vi "gameplay scene.vi"(8 "hold note key":T1, 9 "gameplay info":T2, 10 "chart info":T3, 11 "new picture in":picture) -> (3 "new picture":picture)   [LabVIEW 2023]
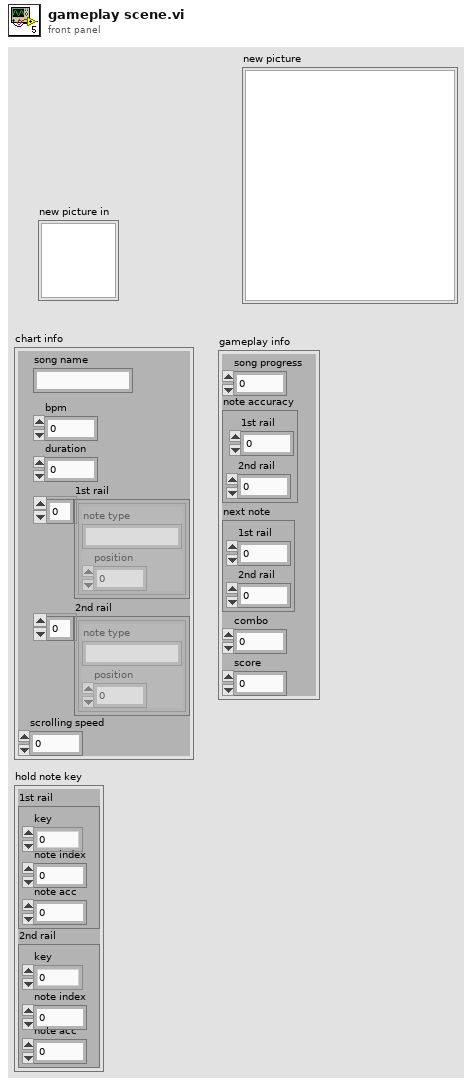
[diagram p1: front panel]
types:
  T1 = cluster{"1st rail":cluster{"key":enum16{"0", "1", "2", "3", "4", "5", "6", "7", "8", "9", "A", "B", "C", "D", "E", "F", "G", "H", "I", "J", "K", "L", "M", "N", "O", "P", "Q", "R", "S", "T", "U", "V", "W", "X", "Y", "Z", "F1", "F2", "F3", "F4", "F5", "F6", "F7", "F8", "F9", "F10", "F11", "F12", "F13", "F14", "F15", "ADD", "BACK", "BACKSLASH", "CAPITAL", "COMMA", "DECIMAL", "DELETE", "DIVIDE", "DOWN", "END", "EQUALS", "ESCAPE", "GRAVE (`)", "HOME", "INSERT", "LBRACKET", "LCONTROL", "LEFT", "L ALT", "LSHIFT", "LWIN", "MINUS", "MULTIPLY", "NEXT", "NUMLOCK", "NUMPAD_0", "NUMPAD_1", "NUMPAD_2", "NUMPAD_3", "NUMPAD_4", "NUMPAD_5", "NUMPAD_6", "NUMPAD_7", "NUMPAD_8", "NUMPAD_9", "PAUSE", "PERIOD", "PRIOR (PG UP)", "RBRACKET", "RCONTROL", "RETURN", "RIGHT", "R ALT", "RSHIFT", "RWIN", "SCROLL", "SEMICOLON", "SLASH", "SPACE", "SUBTRACT", "TAB", "UP", "ENTER (num pad)", "' (quote)"}, "note index":i32, "note acc":i32}, "2nd rail":cluster{"key":enum16{"0", "1", "2", "3", "4", "5", "6", "7", "8", "9", "A", "B", "C", "D", "E", "F", "G", "H", "I", "J", "K", "L", "M", "N", "O", "P", "Q", "R", "S", "T", "U", "V", "W", "X", "Y", "Z", "F1", "F2", "F3", "F4", "F5", "F6", "F7", "F8", "F9", "F10", "F11", "F12", "F13", "F14", "F15", "ADD", "BACK", "BACKSLASH", "CAPITAL", "COMMA", "DECIMAL", "DELETE", "DIVIDE", "DOWN", "END", "EQUALS", "ESCAPE", "GRAVE (`)", "HOME", "INSERT", "LBRACKET", "LCONTROL", "LEFT", "L ALT", "LSHIFT", "LWIN", "MINUS", "MULTIPLY", "NEXT", "NUMLOCK", "NUMPAD_0", "NUMPAD_1", "NUMPAD_2", "NUMPAD_3", "NUMPAD_4", "NUMPAD_5", "NUMPAD_6", "NUMPAD_7", "NUMPAD_8", "NUMPAD_9", "PAUSE", "PERIOD", "PRIOR (PG UP)", "RBRACKET", "RCONTROL", "RETURN", "RIGHT", "R ALT", "RSHIFT", "RWIN", "SCROLL", "SEMICOLON", "SLASH", "SPACE", "SUBTRACT", "TAB", "UP", "ENTER (num pad)", "' (quote)"}, "note index":i32, "note acc":i32}}
  T2 = cluster{"song progress":dbl, "note accuracy":cluster{"1st rail":i32, "2nd rail":i32}, "next note":cluster{"1st rail":i32, "2nd rail":i32}, "combo":i32, "score":i32}
  T3 = cluster{"song name":string, "bpm":i32, "duration":i32, "1st rail":cluster{"note type":string, "position":dbl}[], "2nd rail":cluster{"note type":string, "position":dbl}[], "scrolling speed":dbl}
  T4 = cluster{"Font Name:":string, "Size":i16, "Strikeout?":bool, "Italic?":bool, "Underline?":bool, "Outline?":bool, "Shadow?":bool, "Bold?":bool}
  T5 = enum16{"User-specified Font", "Application Font", "System Font", "Dialog Font"}
  T6 = cluster{"horizontal":enum16{"left", "center", "right"}, "vertical":enum16{"top", "center", "bottom"}}
  T7 = enum16{"0", "1", "2", "3", "4", "5", "6", "7", "8", "9", "A", "B", "C", "D", "E", "F", "G", "H", "I", "J", "K", "L", "M", "N", "O", "P", "Q", "R", "S", "T", "U", "V", "W", "X", "Y", "Z", "F1", "F2", "F3", "F4", "F5", "F6", "F7", "F8", "F9", "F10", "F11", "F12", "F13", "F14", "F15", "ADD", "BACK", "BACKSLASH", "CAPITAL", "COMMA", "DECIMAL", "DELETE", "DIVIDE", "DOWN", "END", "EQUALS", "ESCAPE", "GRAVE (`)", "HOME", "INSERT", "LBRACKET", "LCONTROL", "LEFT", "L ALT", "LSHIFT", "LWIN", "MINUS", "MULTIPLY", "NEXT", "NUMLOCK", "NUMPAD_0", "NUMPAD_1", "NUMPAD_2", "NUMPAD_3", "NUMPAD_4", "NUMPAD_5", "NUMPAD_6", "NUMPAD_7", "NUMPAD_8", "NUMPAD_9", "PAUSE", "PERIOD", "PRIOR (PG UP)", "RBRACKET", "RCONTROL", "RETURN", "RIGHT", "R ALT", "RSHIFT", "RWIN", "SCROLL", "SEMICOLON", "SLASH", "SPACE", "SUBTRACT", "TAB", "UP", "ENTER (num pad)", "' (quote)"}
  T8 = cluster{"Width":u16, "Style":enum32{"Solid", "Dash", "Dot", "DashDot", "DashDotDot"}}
  T9 = cluster{"Width":i16, "Style":enum32{"Solid", "Dash", "Dot", "DashDot", "DashDotDot"}}
  T10 = enum16{"0", "1", "2", "3", "4", "5", "6", "7", "8", "9", "A", "B", "C", "D", "E", "F", "G", "H", "I", "J", "K", "L", "M", "N", "O", "P", "Q", "R", "S", "T", "U", "V", "W", "X", "Y", "Z", "F1", "F2", "F3", "F4", "F5", "F6", "F7", "F8", "F9", "F10", "F11", "F12", "F13", "F14", "F15", "ADD", "BACK", "BACKSLASH", "CAPITAL", "COMMA", "DECIMAL", "DELETE", "DIVIDE", "DOWN", "END", "EQUALS", "ESCAPE", "GRAVE (`)", "HOME", "INSERT", "LBRACKET", "LCONTROL", "LEFT", "L ALT", "LSHIFT", "LWIN", "MINUS", "MULTIPLY", "NEXT", "NUMLOCK", "NUMPAD_0", "NUMPAD_1", "NUMPAD_2", "NUMPAD_3", "NUMPAD_4", "NUMPAD_5", "NUMPAD_6", "NUMPAD_7", "NUMPAD_8", "NUMPAD_9", "PAUSE", "PERIOD", "PRIOR (PG UP)", "RBRACKET", "RCONTROL", "RETURN", "RIGHT", "R ALT", "RSHIFT", "RWIN", "SCROLL", "SEMICOLON", "SLASH", "SPACE", "SUBTRACT", "TAB", "UP", "ENTER (num pad)", "' (quote)"}[]
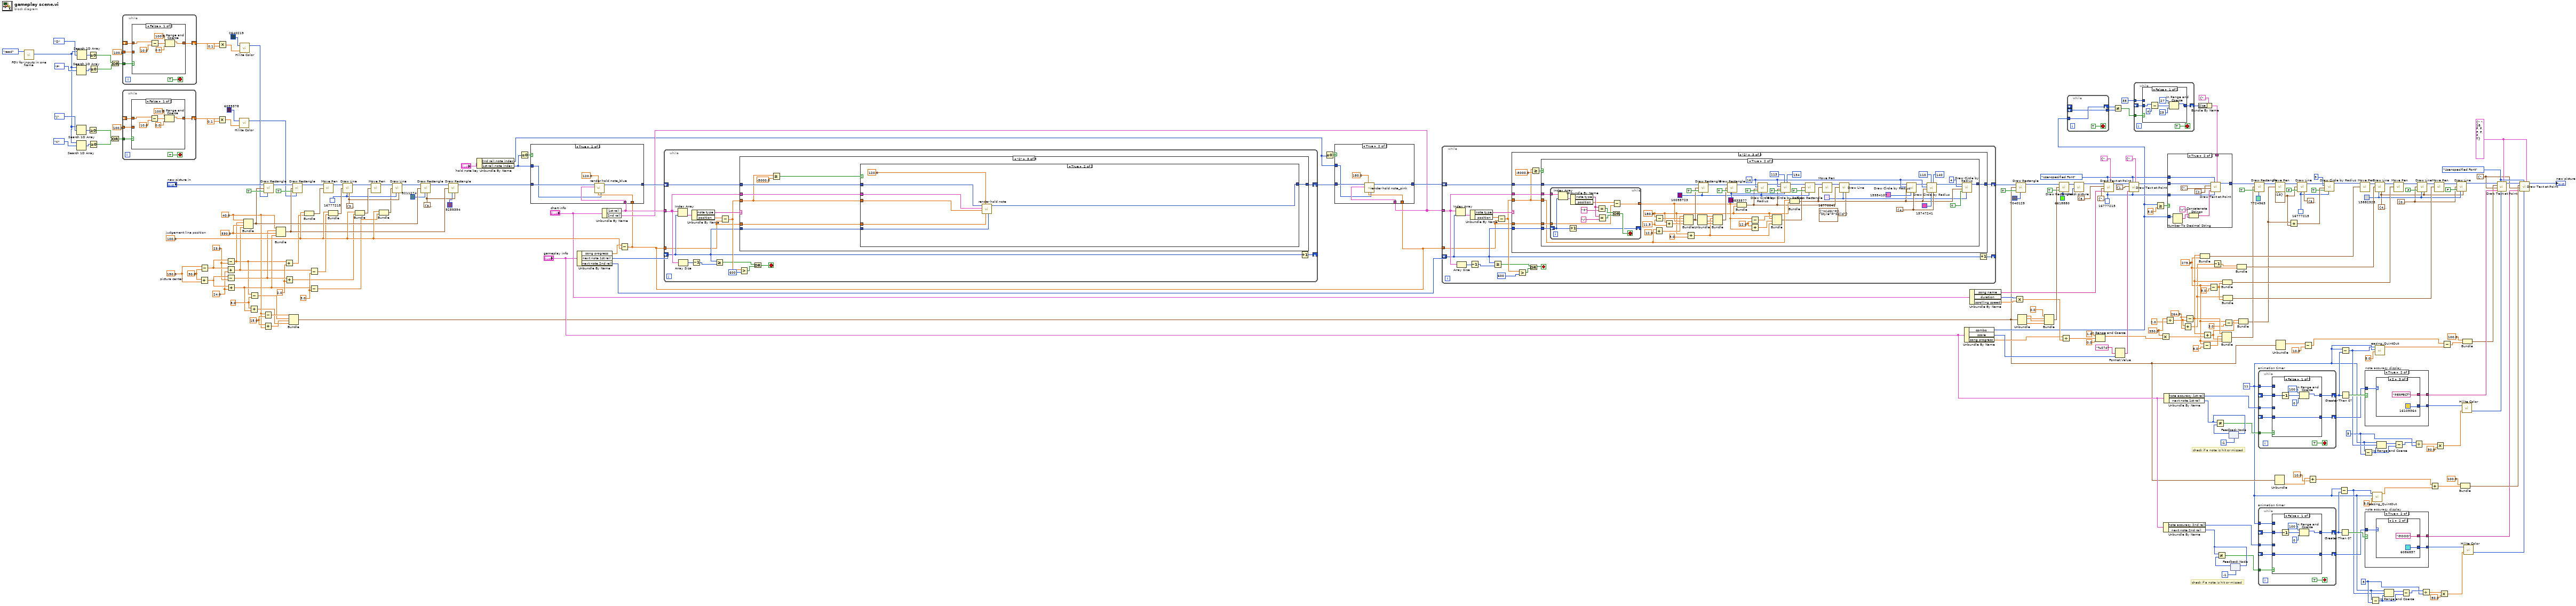
[diagram p0: block diagram]
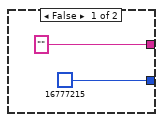
[diagram p2: hidden frame]
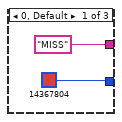
[diagram p3: hidden frame]
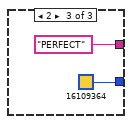
[diagram p4: hidden frame]
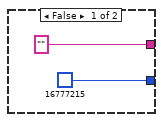
[diagram p6: hidden frame]
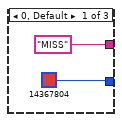
[diagram p7: hidden frame]
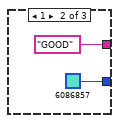
[diagram p8: hidden frame]
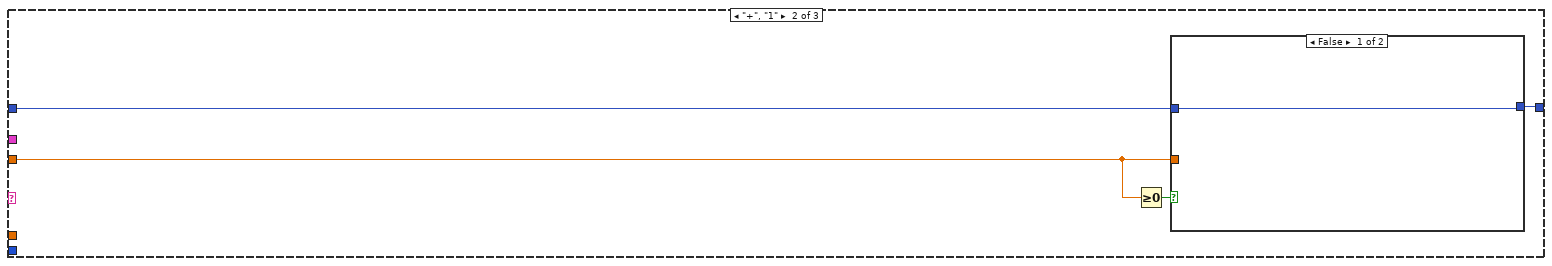
[diagram p17: hidden frame]
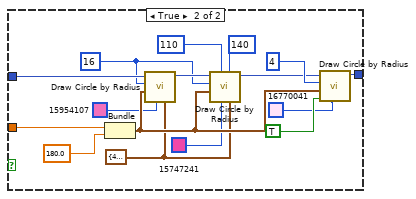
[diagram p18: hidden frame]
diagram:
  w12 = 5
  w39 = 5
  w9 = 11
  w19 = T4 {"Font Name:"=" ", "Size"=18, "Strikeout?"=FALSE, "Italic?"=FALSE, "Underline?"=FALSE, "Outline?"=FALSE, "Shadow?"=FALSE, "Bold?"=TRUE} ("[user-specified font]")
  w20 = T5."User-specified Font" ("desired font(Application)")
  w7 = T6 {"horizontal"=enum."center", "vertical"=enum."center"} ("alignment(left, top)")
  w115 = u32 16777215 ("color(black)")
  w119 = cluster{"x":i16, "y":i16} {"x"=0, "y"=-15} ("end point")
  w139 = cluster{"x":i16, "y":i16} {"x"=0, "y"=12} ("end point")
  w146 = u32 13882323 ("color(black)")
  w138 = T8 {"Width"=4, "Style"=enum."Solid"} ("pen")
  w129 = 275.0
  w160 = 264.0
  w162 = 350.0
  w167 = u32 16777215 ("text color(black)")
  w168 = T5."User-specified Font" ("desired font(Application)")
  w188 = u32 6618880 ("color(black)")
  w201 = 8.0
  w205 = 15.0
  w206 = 24.0
  w207 = 2.0
  w211 = 3.0
  w216 = T9 {"Width"=3, "Style"=enum."Solid"} ("pen")
  w222 = 530.0
  w214 = 23.0
  w228 = 30.0
  w227 = 150.0  # picture center
  w204 = 40.0
  w234 = T8 {"Width"=3, "Style"=enum."Solid"} ("pen")
  w233 = u32 16777215 ("color(black)")
  w231 = 100.0  # judgement line position
  # "check if a note is hit or missed"
  # "check if a note is hit or missed"
  n1 = call "FGV for inputs in one frame.vi"("mode"=enum16{"read", "write"}."read") -> ("read out key"=w74:T10)  [unwired: 10 in]
  n2 = Search 1D Array(1D array=w74, element=T7."K") -> (index of element=w76:i32)  [unwired: 1 in]
  n3 = Search 1D Array(1D array=w74, element=T7."F") -> (index of element=w99:i32)  [unwired: 1 in]
  n4 = Search 1D Array(1D array=w74, element=T7."J") -> (index of element=w75:i32)  [unwired: 1 in]
  n5 = Search 1D Array(1D array=w74, element=T7."D") -> (index of element=w100:i32)  [unwired: 1 in]
  n6 = Greater Or Equal To 0?(x=w75) -> (x >= 0?=w84:bool)
  n7 = Greater Or Equal To 0?(x=w100) -> (x >= 0?=w87:bool)
  n8 = Greater Or Equal To 0?(x=w76) -> (x >= 0?=w85:bool)
  n9 = Greater Or Equal To 0?(x=w99) -> (x >= 0?=w86:bool)
  n10 = Or(x=w84, y=w85) -> (x .or. y?=w83:bool)
  n11 = Or(x=w87, y=w86) -> (x .or. y?=w88:bool)
  n12 = while {
    tunnel: w83 -> [w247]
    tunnel: 100.0 -> [w246]
    shift-right: [w245] -> w78
    shift-left: _ -> [w244]
    stop <- TRUE stop-if-true
    n13 = case shown="False" w247 {
      tunnel: w246 -> [_ w255]
      tunnel: [w250 w255] -> w245
      tunnel: w244 -> [w254 _]
      frame False {
        n14 = Subtract(x=w254, y=10.0) -> (x-y=w252:dbl)
        n15 = In Range and Coerce(upper limit=100.0, x=w252, lower limit=0.0 ("upper limit")) -> (coerced(x)=w250:dbl)  [unwired: 1 out]
      }
      frame True {
      }
    }
  }
  n16 = while {
    tunnel: w88 -> [w259]
    tunnel: 100.0 -> [w258]
    shift-right: [w257] -> w97
    shift-left: _ -> [w256]
    stop <- TRUE stop-if-true
    n17 = case shown="False" w259 {
      tunnel: w258 -> [_ w267]
      tunnel: [w262 w267] -> w257
      tunnel: w256 -> [w266 _]
      frame False {
        n18 = Subtract(x=w266, y=10.0) -> (x-y=w264:dbl)
        n19 = In Range and Coerce(upper limit=100.0, x=w264, lower limit=0.0 ("upper limit")) -> (coerced(x)=w262:dbl)  [unwired: 1 out]
      }
      frame True {
      }
    }
  }
  n20 = Add(x=w228, y=w227) -> (x+y=w225:dbl)
  n21 = Subtract(x=w227, y=w228) -> (x-y=w226:dbl)
  n22 = Multiply(x=w78, y=0.1) -> (x*y=w80:dbl)
  n23 = Multiply(x=w97, y=0.1) -> (x*y=w95:dbl)
  n24 = Subtract(x=w226, y=w214) -> (x-y=w196:dbl)
  n25 = Add(x=w226, y=w206) -> (x+y=w200:dbl)
  n26 = Subtract(x=w225, y=w214) -> (x-y=w209:dbl)
  n27 = Add(x=w225, y=w206) -> (x+y=w199:dbl)
  n28 = call <vilib>:"Hilite Color.vi"("Percentage(30)"=w80, "Color In"=u32 6039378 ("color(black)")) -> ("Hilite"=w72:u32)  [unwired: 1 out]
  n29 = call <vilib>:"Hilite Color.vi"("Percentage(30)"=w95, "Color In"=u32 2640219 ("color(black)")) -> ("Hilite"=w92:u32)  [unwired: 1 out]
  n30 = Bundle(w204, w196, w222, w200) -> (w219:cluster{dbl, dbl, dbl, dbl})  [unwired: 1 in]
  n31 = Add(x=w201, y=w199) -> (x+y=w197:dbl)
  n32 = Subtract(x=w196, y=w201) -> (x-y=w198:dbl)
  n33 = Subtract(x=w204, y=w205) -> (x-y=w203:dbl)
  n34 = Add(x=w205, y=w204) -> (x+y=w202:dbl)
  n35 = call <vilib>:"Draw Rectangle.vi"("picture"="new picture in", "rect"=w219, "fill?(F)"=TRUE, "color(black)"=w92) -> ("new picture"=w224:picture)  [unwired: 5 in]
  n36 = Bundle(w204, w209, w222, w199) -> (w217:cluster{dbl, dbl, dbl, dbl})  [unwired: 1 in]
  n37 = Add(x=w196, y=w207) -> (x+y=w210:dbl)
  n38 = Add(x=w209, y=w207) -> (x+y=w208:dbl)
  n39 = Bundle(w203, w198, w202, w197) -> (w29:cluster{dbl, dbl, dbl, dbl})  [unwired: 1 in]
  n40 = call <vilib>:"Draw Rectangle.vi"("picture"=w224, "rect"=w217, "fill?(F)"=TRUE, "color(black)"=w72) -> ("new picture"=w221:picture)  [unwired: 5 in]
  n41 = Bundle("judgement line position"=w231, w210) -> (w240:cluster{"judgement line position":dbl, dbl})  [unwired: 1 in]
  n42 = Subtract(x=w200, y=w211) -> (x-y=w213:dbl)
  n43 = Subtract(x=w199, y=w211) -> (x-y=w212:dbl)
  n44 = call <vilib>:"Move Pen.vi"("new position"=w240, "picture"=w221) -> ("new picture"=w239:picture)  [unwired: 3 in]
  n45 = Bundle("judgement line position"=w231, w213) -> (w238:cluster{"judgement line position":dbl, dbl})  [unwired: 1 in]
  n46 = call <vilib>:"Draw Line.vi"("picture"=w239, "end point"=w238, "color(black)"=w233, "pen"=w234) -> ("new picture"=w237:picture)  [unwired: 5 in]
  n47 = Bundle("judgement line position"=w231, w208) -> (w236:cluster{"judgement line position":dbl, dbl})  [unwired: 1 in]
  n48 = call <vilib>:"Move Pen.vi"("new position"=w236, "picture"=w237) -> ("new picture"=w235:picture)  [unwired: 3 in]
  n49 = Bundle("judgement line position"=w231, w212) -> (w232:cluster{"judgement line position":dbl, dbl})  [unwired: 1 in]
  n50 = call <vilib>:"Draw Line.vi"("picture"=w235, "end point"=w232, "color(black)"=w233, "pen"=w234) -> ("new picture"=w220:picture)  [unwired: 5 in]
  n51 = call <vilib>:"Draw Rectangle.vi"("picture"=w220, "rect"=w219, "color(black)"=u32 5211274, "pen"=w216) -> ("new picture"=w218:picture)  [unwired: 5 in]
  n52 = call <vilib>:"Draw Rectangle.vi"("picture"=w218, "rect"=w217, "color(black)"=u32 9259394, "pen"=w216) -> ("new picture"=w112:picture)  [unwired: 5 in]
  n53 = Unbundle By Name("hold note key") -> ("2nd rail.note index"=w101:i32, "1st rail.note index"=w107:i32)
  n54 = Greater Or Equal To 0?(x=w107) -> (x >= 0?=w108:bool)
  n55 = Unbundle By Name("gameplay info") -> ("song progress"=w241:dbl, "next note.1st rail"=w243:i32, "next note.2nd rail"=w242:i32)
  n56 = Unbundle By Name("chart info") -> ("1st rail"=w109:cluster{"note type":string, "position":dbl}[], "2nd rail"=w104:cluster{"note type":string, "position":dbl}[])
  n57 = Subtract(x=w241, y=w231) -> (x-y=w103:dbl)
  n58 = case shown="True" w108 {
    tunnel: w112 -> [w268 w272]
    tunnel: [w268 w273] -> w111
    tunnel: w109 -> [_ w271]
    tunnel: w103 -> [_ w270]
    tunnel: w107 -> [_ w269]
    frame False {
    }
    frame True {
      n59 = call "render hold note_blue.vi"("head index"=w269, "progress"=w270, "y-center"=120.0, "rail"=w271, "new picture in"=w272) -> ("new picture out"=w273:picture)  [unwired: 6 in]
    }
  }
  n60 = while {
    tunnel: w109 -> [w277]
    tunnel: w103 -> [w275]
    shift-right: [w290] -> _
    shift-left: w243 -> [w276]
    shift-right: [w285] -> w106
    shift-left: w111 -> [w284]
    stop <- w278 stop-if-true
    n61 = Index Array(array=w277, index=w276) -> (element=w289:cluster{"note type":string, "position":dbl})
    n62 = Array Size(array=w277) -> (size(s)=w282:i32)
    n63 = Decrement(x=w282) -> (x-1=w281:i32)
    n64 = Unbundle By Name(w289) -> ("note type"=w286:string, "position"=w288:dbl)
    n65 = Greater Or Equal?(x=w276, y=w281) -> (x >= y?=w279:bool)
    n66 = Subtract(x=w288, y=w275) -> (x-y=w283:dbl)
    n67 = Greater?(x=w283, y=600) -> (0:w280:bool)
    n68 = case shown="\"2\"" w286 {
      tunnel: [w291 w294 w320] -> w285
      tunnel: w284 -> [w291 w295 w317]
      tunnel: w283 -> [_ w292 w313]
      tunnel: w277 -> [_ _ w319]
      tunnel: w276 -> [_ _ w318]
      tunnel: w275 -> [_ _ w315]
      frame "0", Default {
      }
      frame "+", "1" {
        n69 = Greater Or Equal To 0?(x=w292) -> (x >= 0?=w293:bool)
        n70 = case shown="True" w293 {
          tunnel: w295 -> [w296 w312]
          tunnel: w292 -> [_ w310]
          tunnel: [w296 w308] -> w294
          frame False {
          }
          frame True {
            w301 = T8 {"Width"=4, "Style"=enum."Solid"} ("pen")
            w304 = i16 16 ("radius")
            n71 = Bundle(w310, 120.0) -> (w303:cluster{dbl, dbl})  [unwired: 1 in]
            n72 = call <vilib>:"Draw Circle by Radius.vi"("pen"=w301, "color(black)"=u32 7464690, "pixel center"=w303, "radius"=w304, "picture"=w312) -> ("new picture"=w306:picture)  [unwired: 6 in]
            n73 = call <vilib>:"Draw Circle by Radius.vi"("pen"=w301, "arc size(360)"=i16 140 ("radius"), "color(black)"=u32 2873836, "start angle(0)"=i16 110 ("radius"), "pixel center"=w303, "radius"=w304, "picture"=w306) -> ("new picture"=w305:picture)  [unwired: 4 in]
            n74 = call <vilib>:"Draw Circle by Radius.vi"("color(black)"=u32 14942206, "fill?(F)"=TRUE, "pixel center"=w303, "radius"=i16 4, "picture"=w305) -> ("new picture"=w308:picture)  [unwired: 6 in]
          }
        }
      }
      frame "2" {
        n75 = Greater Or Equal?(x=w313, y=-5000.0) -> (x >= y?=w316:bool)
        n76 = case shown="True" w316 {
          tunnel: [w321 w328] -> w320
          tunnel: w319 -> [_ w327]
          tunnel: w318 -> [_ w326]
          tunnel: w315 -> [_ w325]
          tunnel: w317 -> [w321 w324]
          tunnel: w313 -> [_ w323]
          frame False {
          }
          frame True {
            n77 = call "render hold note.vi"("head index"=w326, "progress"=w325, "y-center"=120.0, "head position"=w323, "rail"=w327, "new picture in"=w324) -> ("new picture out"=w328:picture)  [unwired: 5 in]
          }
        }
      }
    }
    n78 = Or(x=w279, y=w280) -> (x .or. y?=w278:bool)
    n79 = Increment(x=w276) -> (x+1=w290:i32)
  }
  n80 = Greater Or Equal To 0?(x=w101) -> (x >= 0?=w102:bool)
  n81 = case shown="True" w102 {
    tunnel: w106 -> [w329 w334]
    tunnel: [w329 w333] -> w105
    tunnel: w104 -> [_ w335]
    tunnel: w103 -> [_ w331]
    tunnel: w101 -> [_ w330]
    frame False {
    }
    frame True {
      n82 = call "render hold note_pink.vi"("head index"=w330, "progress"=w331, "y-center"=180.0, "rail"=w335, "new picture in"=w334) -> ("new picture out"=w333:picture)  [unwired: 6 in]
    }
  }
  n83 = while {
    tunnel: w104 -> [w338]
    tunnel: w103 -> [w336]
    shift-right: [w351] -> _
    shift-left: w242 -> [w337]
    shift-right: [w346] -> w193
    shift-left: w105 -> [w345]
    stop <- w339 stop-if-true
    n84 = Index Array(array=w338, index=w337) -> (element=w350:cluster{"note type":string, "position":dbl})
    n85 = Array Size(array=w338) -> (size(s)=w343:i32)
    n86 = Decrement(x=w343) -> (x-1=w342:i32)
    n87 = Unbundle By Name(w350) -> ("note type"=w347:string, "position"=w349:dbl)
    n88 = Greater Or Equal?(x=w337, y=w342) -> (x >= y?=w340:bool)
    n89 = Subtract(x=w349, y=w336) -> (x-y=w344:dbl)
    n90 = case shown="\"2\"" w347 {
      tunnel: [w352 w355 w381] -> w346
      tunnel: w345 -> [w352 w356 w377]
      tunnel: w344 -> [_ w353 w374]
      tunnel: w338 -> [_ _ w380]
      tunnel: w337 -> [_ _ w379]
      tunnel: w336 -> [_ _ w378]
      frame "0", Default {
      }
      frame "+", "1" {
        n91 = Greater Or Equal To 0?(x=w353) -> (x >= 0?=w354:bool)
        n92 = case shown="False" w354 {
          tunnel: w356 -> [w357 w373]
          tunnel: w353 -> [_ w371]
          tunnel: [w357 w369] -> w355
          frame False {
          }
          frame True {
            w362 = T8 {"Width"=4, "Style"=enum."Solid"} ("pen")
            w365 = i16 16 ("radius")
            n93 = Bundle(w371, 180.0) -> (w364:cluster{dbl, dbl})  [unwired: 1 in]
            n94 = call <vilib>:"Draw Circle by Radius.vi"("pen"=w362, "color(black)"=u32 15954107, "pixel center"=w364, "radius"=w365, "picture"=w373) -> ("new picture"=w367:picture)  [unwired: 6 in]
            n95 = call <vilib>:"Draw Circle by Radius.vi"("pen"=w362, "arc size(360)"=i16 140 ("radius"), "color(black)"=u32 15747241, "start angle(0)"=i16 110 ("radius"), "pixel center"=w364, "radius"=w365, "picture"=w367) -> ("new picture"=w366:picture)  [unwired: 4 in]
            n96 = call <vilib>:"Draw Circle by Radius.vi"("color(black)"=u32 16770041, "fill?(F)"=TRUE, "pixel center"=w364, "radius"=i16 4, "picture"=w366) -> ("new picture"=w369:picture)  [unwired: 6 in]
          }
        }
      }
      frame "2" {
        n97 = Greater Or Equal?(x=w374, y=-5000.0) -> (x >= y?=w376:bool)
        n98 = case shown="True" w376 {
          tunnel: [w382 w435] -> w381
          tunnel: w380 -> [_ w427]
          tunnel: w379 -> [_ w426]
          tunnel: w378 -> [_ w425]
          tunnel: w377 -> [w382 w424]
          tunnel: w374 -> [_ w423]
          frame False {
          }
          frame True {
            w396 = 12.0 ("y")
            w404 = u32 9833577 ("color(black)")
            w384 = u32 16770041 ("color(black)")
            w397 = u32 10095723 ("color(black)")
            w419 = 11.5 ("y")
            w431 = T8 {"Width"=4, "Style"=enum."Solid"} ("pen")
            w391 = 180.0
            w400 = i16 16 ("radius")
            n99 = while {
              tunnel: w427 -> [w449]
              shift-right: [w440] -> _
              shift-left: w426 -> [w441]
              tunnel: w425 -> [w439]
              tunnel: [w437] -> w395
              stop <- w442 stop-if-true
              n100 = Index Array(array=w449, index=w441) -> (element=w448:cluster{"note type":string, "position":dbl})
              n101 = Increment(x=w441) -> (x+1=w440:i32)
              n102 = Unbundle By Name(w448) -> ("note type"=w445:string, "position"=w438:dbl)
              n103 = Equal?(x=w445, y="+") -> (x = y?=w447:bool)
              n104 = Equal?(x=w445, y="-") -> (x = y?=w446:bool)
              n105 = Or(x=w447, y=w446) -> (x .or. y?=w442:bool)
              n106 = Subtract(x=w438, y=w439) -> (x-y=w437:dbl)
            }
            n107 = Add(x=w423, y=12.0) -> (x+y=w421:dbl)
            n108 = Subtract(x=w391, y=w419) -> (x-y=w420:dbl)
            n109 = Add(x=w391, y=w419) -> (x+y=w418:dbl)
            n110 = Bundle(w421, w420, w395, w418) -> (w411:cluster{dbl, dbl, dbl, dbl})  [unwired: 1 in]
            n111 = Add(x=w391, y=5.0) -> (x+y=w392:dbl)
            n112 = Unbundle(w411) -> (w410:dbl, w409:dbl, w408:dbl)  [unwired: 1 out]
            n113 = call <vilib>:"Draw Rectangle.vi"("picture"=w424, "rect"=w411, "fill?(F)"=TRUE, "color(black)"=w397) -> ("new picture"=w414:picture)  [unwired: 5 in]
            n114 = Bundle(w410, w392, w409, w408) -> (w406:cluster{dbl, dbl, dbl, dbl})  [unwired: 1 in]
            n115 = call <vilib>:"Draw Rectangle.vi"("picture"=w414, "rect"=w406, "fill?(F)"=TRUE, "color(black)"=w404) -> ("new picture"=w413:picture)  [unwired: 5 in]
            n116 = Bundle(w395, w391) -> (w386:cluster{dbl, dbl})  [unwired: 1 in]
            n117 = Subtract(x=w395, y=w396) -> (x-y=w394:dbl)
            n118 = Add(x=w396, y=w395) -> (x+y=w393:dbl)
            n119 = call <vilib>:"Draw Circle by Radius.vi"("color(black)"=w397, "fill?(F)"=TRUE, "pixel center"=w386, "radius"=w400, "picture"=w413) -> ("new picture"=w405:picture)  [unwired: 6 in]
            n120 = Bundle(w394, w391, w393, w392) -> (w390:cluster{dbl, dbl, dbl, dbl})  [unwired: 1 in]
            n121 = call <vilib>:"Draw Circle by Radius.vi"("arc size(360)"=i16 134 ("radius"), "color(black)"=w404, "start angle(0)"=i16 113 ("radius"), "fill?(F)"=TRUE, "pixel center"=w386, "radius"=w400, "picture"=w405) -> ("new picture"=w399:picture)  [unwired: 4 in]
            n122 = Bundle(w423, w391) -> (w388:cluster{dbl, dbl})  [unwired: 1 in]
            n123 = call <vilib>:"Draw Rectangle.vi"("picture"=w399, "rect"=w390, "fill?(F)"=TRUE, "color(black)"=w397) -> ("new picture"=w389:picture)  [unwired: 5 in]
            n124 = call <vilib>:"Move Pen.vi"("new position"=w388, "picture"=w389) -> ("new picture"=w387:picture)  [unwired: 3 in]
            n125 = call <vilib>:"Draw Line.vi"("picture"=w387, "end point"=w386, "color(black)"=w384, "pen"=T8 {"Width"=2, "Style"=enum."Solid"}) -> ("new picture"=w385:picture)  [unwired: 5 in]
            n126 = call <vilib>:"Draw Circle by Radius.vi"("pen"=w431, "color(black)"=u32 15954107, "pixel center"=w388, "radius"=w400, "picture"=w385) -> ("new picture"=w433:picture)  [unwired: 6 in]
            n127 = call <vilib>:"Draw Circle by Radius.vi"("pen"=w431, "arc size(360)"=i16 140 ("radius"), "color(black)"=u32 15747241, "start angle(0)"=i16 110 ("radius"), "pixel center"=w388, "radius"=w400, "picture"=w433) -> ("new picture"=w432:picture)  [unwired: 4 in]
            n128 = call <vilib>:"Draw Circle by Radius.vi"("color(black)"=w384, "fill?(F)"=TRUE, "pixel center"=w388, "radius"=i16 4, "picture"=w432) -> ("new picture"=w435:picture)  [unwired: 6 in]
          }
        }
      }
    }
    n129 = Greater?(x=w344, y=600) -> (0:w341:bool)
    n130 = Or(x=w340, y=w341) -> (x .or. y?=w339:bool)
    n131 = Increment(x=w337) -> (x+1=w351:i32)
  }
  n132 = Unbundle By Name("gameplay info") -> ("combo"=w69:i32, "score"=w174:i32, "song progress"=w163:dbl)
  n133 = Unbundle By Name("chart info") -> ("song name"=w179:string, "duration"=w165:i32, "scrolling speed"=w166:dbl)
  n134 = Multiply(x=w165, y=w166) -> (x*y=w164:dbl)
  n135 = call <vilib>:"Draw Rectangle.vi"("picture"=w193, "rect"=w29, "fill?(F)"=TRUE, "color(black)"=u32 7040129) -> ("new picture"=w191:picture)  [unwired: 5 in]
  n136 = Unbundle(w29) -> (w192:dbl, w185:dbl, w184:dbl)  [unwired: 1 out]
  n137 = Bundle(0.0, w185, w192, w184) -> (w190:cluster{dbl, dbl, dbl, dbl})  [unwired: 1 in]
  n138 = call <vilib>:"Draw Rectangle.vi"("picture"=w191, "rect"=w190, "fill?(F)"=TRUE, "color(black)"=w188) -> ("new picture"=w187:picture)  [unwired: 5 in]
  n139 = Divide(x=w163, y=w164) -> (x/y=w145:dbl)
  n140 = while {
    shift-right: [w451] -> w67
    shift-left: _ -> [_]
    shift-left: _ -> [w450]
    tunnel: w69 -> [w451]
    tunnel: [w450] -> w68
    stop <- TRUE stop-if-true
  }
  n141 = call "mask picture.vi"("mask color"=w188, "new picture in"=w187) -> ("new picture out"=w182:picture)  [unwired: 9 in]
  n142 = In Range and Coerce(upper limit=1.0, x=w145, lower limit=0.0) -> (coerced(x)=w144:dbl)  [unwired: 1 out]
  n143 = call <vilib>:"Draw Text at Point.vi"("[user-specified font]"=T4 {"Font Name:"=" ", "Size"=13, "Strikeout?"=FALSE, "Italic?"=FALSE, "Underline?"=FALSE, "Outline?"=FALSE, "Shadow?"=FALSE, "Bold?"=TRUE}, "text color(black)"=w167, "desired font(Application)"=w168, "text"=w179, "alignment(left, top)"=T6 {"horizontal"=enum."right", "vertical"=enum."top"}, "origin"=cluster{"x":i16, "y":i16} {"x"=510, "y"=5}, "picture"=w182) -> ("new picture"=w177:picture)  [unwired: 3 in, 1 out]
  n144 = Not Equal?(x=w67, y=w68) -> (x != y?=w66:bool)
  n145 = Format Value(format string="%07d", value (0)=w174) -> (output string=w172:string)  [unwired: 1 in]
  n146 = call <vilib>:"Draw Text at Point.vi"("[user-specified font]"=T4 {"Font Name:"=" ", "Size"=21, "Strikeout?"=FALSE, "Italic?"=FALSE, "Underline?"=FALSE, "Outline?"=FALSE, "Shadow?"=FALSE, "Bold?"=TRUE}, "text color(black)"=w167, "desired font(Application)"=w168, "text"=w172, "origin"=cluster{"x":i16, "y":i16} {"x"=10, "y"=5}, "picture"=w177) -> ("new picture"=w169:picture)  [unwired: 4 in, 1 out]
  n147 = while {
    tunnel: w66 -> [w456]
    tunnel: 35 -> [w455]
    shift-right: [w454] -> w64
    shift-left: _ -> [w453]
    stop <- TRUE stop-if-true
    n148 = case shown="False" w456 {
      tunnel: w455 -> [_ w464]
      tunnel: [w463 w464] -> w454
      tunnel: w453 -> [w459 _]
      frame False {
        n149 = Subtract(x=w459, y=4) -> (x-y=w462:i32)
        n150 = In Range and Coerce(upper limit=27, x=w462, lower limit=25 ("upper limit")) -> (coerced(x)=w463:i32)  [unwired: 1 out]
      }
      frame True {
      }
    }
  }
  n151 = Greater Or Equal?(x=w69, y=5.0) -> (x >= y?=w171:bool)
  n152 = Multiply(x=w162, y=w144) -> (x*y=w137:dbl)
  n153 = Unbundle By Name("gameplay info") -> ("note accuracy.2nd rail"=w30:i32, "next note.2nd rail"=w32:i32)
  n154 = Unbundle By Name("gameplay info") -> ("note accuracy.1st rail"=w57:i32, "next note.1st rail"=w53:i32)
  n155 = Divide(x=w162, y=2.0) -> (x/y=w159:dbl)
  n156 = Add(x=w159, y=w160) -> (x+y=w113:dbl)
  n157 = Subtract(x=w160, y=w159) -> (x-y=w130:dbl)
  n158 = Bundle By Name(cluster=T4 {"Font Name:"=" ", "Size"=25, "Strikeout?"=FALSE, "Italic?"=FALSE, "Underline?"=FALSE, "Outline?"=FALSE, "Shadow?"=FALSE, "Bold?"=TRUE} ("[user-specified font]"), "Size"=w64) -> (w71:T4)
  n159 = case shown="True" w171 {
    tunnel: w169 -> [w465 w476]
    tunnel: [w465 w475] -> w136
    tunnel: w69 -> [_ w473]
    tunnel: w168 -> [_ w474]
    tunnel: w167 -> [_ w469]
    tunnel: w71 -> [_ w466]
    frame False {
    }
    frame True {
      n160 = Number To Decimal String(number=w473) -> (decimal integer string=w472:string)  [unwired: 1 in]
      n161 = Concatenate Strings(w472, "x") -> (w470:string)
      n162 = call <vilib>:"Draw Text at Point.vi"("[user-specified font]"=w466, "text color(black)"=w469, "desired font(Application)"=w474, "text"=w470, "alignment(left, top)"=T6 {"horizontal"=enum."center", "vertical"=enum."center"}, "origin"=cluster{"x":i16, "y":i16} {"x"=264, "y"=50}, "picture"=w476) -> ("new picture"=w475:picture)  [unwired: 3 in, 1 out]
    }
  }
  n163 = Bundle(w130, w129) -> (w141:cluster{dbl, dbl})  [unwired: 1 in]
  n164 = Subtract(x=w129, y=8.0) -> (x-y=w133:dbl)
  n165 = Add(x=w130, y=w137) -> (x+y=w127:dbl)
  n166 = Subtract(x=w129, y=9.0) -> (x-y=w151:dbl)
  n167 = Decrement(x=w113) -> (x-1=w114:dbl)
  n168 = Bundle(w130, w133, w127, w129) -> (w132:cluster{dbl, dbl, dbl, dbl})  [unwired: 1 in]
  n169 = Bundle(w130, w151) -> (w154:cluster{dbl, dbl})  [unwired: 1 in]
  n170 = Bundle(w113, w151) -> (w150:cluster{dbl, dbl})  [unwired: 1 in]
  n171 = Subtract(x=w129, y=3.0 ("x")) -> (x-y=w128:dbl)
  n172 = feedback #1(-1 ("1st rail")) -> (w54:i32)
  n173 = Not Equal?(x=w53, y=w54) -> (x != y?=w52:bool)
  n174 = feedback-in #1(w53) -> ()
  n175 = feedback #2(-1 ("1st rail")) -> (w34:i32)
  n176 = Not Equal?(x=w32, y=w34) -> (x != y?=w31:bool)
  n177 = feedback-in #2(w32) -> ()
  n178 = Bundle(w114, w129) -> (w157:cluster{dbl, dbl})  [unwired: 1 in]
  n179 = Bundle(w127, w128) -> (w120:cluster{dbl, dbl})  [unwired: 1 in]
  n180 = call <vilib>:"Draw Rectangle.vi"("picture"=w136, "rect"=w132, "fill?(F)"=TRUE, "color(black)"=u32 7724963) -> ("new picture"=w131:picture)  [unwired: 5 in]
  n181 = while "animation timer" {
    tunnel: w52 -> [w481]
    tunnel: w9 -> [w483]
    shift-right: [w482] -> w51
    shift-left: _ -> [w480]
    tunnel: w57 -> [w479]
    shift-right: [w478] -> w56
    shift-left: _ -> [w477]
    stop <- TRUE stop-if-true
    n182 = case shown="False" w481 {
      tunnel: w483 -> [_ w492]
      tunnel: [w486 w492] -> w482
      tunnel: w480 -> [w490 _]
      tunnel: w479 -> [_ w491]
      tunnel: [w485 w491] -> w478
      tunnel: w477 -> [w485 _]
      frame False {
        n183 = Decrement(x=w490) -> (x-1=w489:i32)
        n184 = In Range and Coerce(upper limit=100, x=w489, lower limit=0 ("upper limit")) -> (coerced(x)=w486:i32)  [unwired: 1 out]
      }
      frame True {
      }
    }
  }
  n185 = while "animation timer" {
    tunnel: w31 -> [w497]
    tunnel: w9 -> [w499]
    shift-right: [w498] -> w18
    shift-left: _ -> [w496]
    tunnel: w30 -> [w495]
    shift-right: [w494] -> w16
    shift-left: _ -> [w493]
    stop <- TRUE stop-if-true
    n186 = case shown="False" w497 {
      tunnel: w499 -> [_ w508]
      tunnel: [w502 w508] -> w498
      tunnel: w496 -> [w506 _]
      tunnel: w495 -> [_ w507]
      tunnel: [w501 w507] -> w494
      tunnel: w493 -> [w501 _]
      frame False {
        n187 = Decrement(x=w506) -> (x-1=w505:i32)
        n188 = In Range and Coerce(upper limit=100, x=w505, lower limit=0 ("upper limit")) -> (coerced(x)=w502:i32)  [unwired: 1 out]
      }
      frame True {
      }
    }
  }
  n189 = Unbundle(w29) -> (w28:dbl)  [unwired: 3 out]
  n190 = call <vilib>:"Move Pen.vi"("new position"=w120, "picture"=w131) -> ("new picture"=w126:picture)  [unwired: 3 in]
  n191 = Unbundle(w29) -> (w60:dbl)  [unwired: 3 out]
  n192 = Add(x=w120, y=w119) -> (x+y=w118:cluster{dbl, dbl})
  n193 = call <vilib>:"Draw Line.vi"("picture"=w126, "end point"=w119, "absolute coordinates?(T)"=FALSE, "color(black)"=w115, "pen"=T8 {"Width"=3, "Style"=enum."Solid"}) -> ("new picture"=w122:picture)  [unwired: 4 in]
  n194 = Subtract(x=w60, y=10.0) -> (x-y=w48:dbl)
  n195 = Add(x=w28, y=10.0) -> (x+y=w25:dbl)
  n196 = call <vilib>:"Draw Circle by Radius.vi"("color(black)"=w115, "fill?(F)"=TRUE, "pixel center"=w118, "radius"=i16 3, "picture"=w122) -> ("new picture"=w121:picture)  [unwired: 6 in]
  n197 = Subtract(x=w9, y=w18) -> (x-y=w8:i32)
  n198 = Greater Than 0?(x=w18) -> (x > 0?=w17:bool)
  n199 = Subtract(x=w9, y=w51) -> (x-y=w40:i32)
  n200 = Greater Than 0?(x=w51) -> (x > 0?=w59:bool)
  n201 = call <vilib>:"Move Pen.vi"("new position"=w141, "picture"=w121) -> ("new picture"=w158:picture)  [unwired: 3 in]
  n202 = Subtract(x=w9, y=w39) -> (x-y=w38:i32)
  n203 = case "note accuracy display" shown="True" w59 {
    tunnel: w56 -> [_ w513]
    tunnel: ["" w512] -> w58
    tunnel: [u32 16777215 ("text color(black)") w511] -> w45
    frame False {
    }
    frame True {
      n204 = case shown="2" w513 {
        tunnel: ["MISS" "GOOD" "PERFECT"] -> w512
        tunnel: [u32 14367804 ("text color(black)") u32 6086857 ("text color(black)") u32 16109364 ("text color(black)")] -> w511
        frame 0, Default {
        }
        frame 1 {
        }
        frame 2 {
        }
      }
    }
  }
  n205 = case "note accuracy display" shown="True" w17 {
    tunnel: w16 -> [_ w524]
    tunnel: ["" w523] -> w5
    tunnel: [u32 16777215 ("text color(black)") w522] -> w4
    frame False {
    }
    frame True {
      n206 = case shown="1" w524 {
        tunnel: ["MISS" "GOOD" "PERFECT"] -> w523
        tunnel: [u32 14367804 ("text color(black)") u32 6086857 ("text color(black)") u32 16109364 ("text color(black)")] -> w522
        frame 0, Default {
        }
        frame 1 {
        }
        frame 2 {
        }
      }
    }
  }
  n207 = Subtract(x=w9, y=w12) -> (x-y=w13:i32)
  n208 = call "easing_QuintOut.vi"("distance"=5.0 ("y"), "interval (10 ms)"=w9, "time"=w8) -> ("current pos"=w24:dbl)  [unwired: 8 in]
  n209 = call <vilib>:"Draw Line.vi"("picture"=w158, "end point"=w157, "color(black)"=w146, "pen"=w138) -> ("new picture"=w156:picture)  [unwired: 5 in]
  n210 = call "easing_QuintOut.vi"("distance"=5.0 ("y"), "interval (10 ms)"=w9, "time"=w40) -> ("current pos"=w47:dbl)  [unwired: 8 in]
  n211 = In Range and Coerce(upper limit=w9, x=w40, lower limit=w38) -> (coerced(x)=w37:i32)  [unwired: 1 out]
  n212 = In Range and Coerce(upper limit=w9, x=w8, lower limit=w13) -> (coerced(x)=w14:i32)  [unwired: 1 out]
  n213 = call <vilib>:"Move Pen.vi"("new position"=w154, "picture"=w156) -> ("new picture"=w153:picture)  [unwired: 3 in]
  n214 = Subtract(x=w37, y=w38) -> (x-y=w36:i32)
  n215 = Subtract(x=w14, y=w13) -> (x-y=w15:i32)
  n216 = Divide(x=w36, y=w39) -> (x/y=w44:dbl)
  n217 = call <vilib>:"Draw Line.vi"("picture"=w153, "end point"=w139, "absolute coordinates?(T)"=FALSE, "color(black)"=w146, "pen"=w138) -> ("new picture"=w149:picture)  [unwired: 4 in]
  n218 = Divide(x=w15, y=w12) -> (x/y=w10:dbl)
  n219 = Add(x=w25, y=w24) -> (x+y=w22:dbl)
  n220 = call <vilib>:"Move Pen.vi"("new position"=w150, "picture"=w149) -> ("new picture"=w148:picture)  [unwired: 3 in]
  n221 = Multiply(x=w44, y=50.0) -> (x*y=w42:dbl)
  n222 = Multiply(x=w10, y=50.0) -> (x*y=w2:dbl)
  n223 = Subtract(x=w48, y=w47) -> (x-y=w49:dbl)
  n224 = call <vilib>:"Draw Line.vi"("picture"=w148, "end point"=w139, "absolute coordinates?(T)"=FALSE, "color(black)"=w146, "pen"=w138) -> ("new picture"=w63:picture)  [unwired: 4 in]
  n225 = Bundle("y"=100.0, w22) -> (w6:cluster{"y":dbl, dbl})  [unwired: 1 in]
  n226 = call <vilib>:"Hilite Color.vi"("Percentage(30)"=w42, "Color In"=w45) -> ("Shadow"=w41:u32)  [unwired: 1 out]
  n227 = Bundle("y"=100.0, w49) -> (w46:cluster{"y":dbl, dbl})  [unwired: 1 in]
  n228 = call <vilib>:"Hilite Color.vi"("Percentage(30)"=w2, "Color In"=w4) -> ("Shadow"=w3:u32)  [unwired: 1 out]
  n229 = call <vilib>:"Draw Text at Point.vi"("[user-specified font]"=w19, "text color(black)"=w41, "desired font(Application)"=w20, "text"=w58, "alignment(left, top)"=w7, "origin"=w46, "picture"=w63) -> ("new picture"=w21:picture)  [unwired: 3 in, 1 out]
  n230 = call <vilib>:"Draw Text at Point.vi"("[user-specified font]"=w19, "text color(black)"=w3, "desired font(Application)"=w20, "text"=w5, "alignment(left, top)"=w7, "origin"=w6, "picture"=w21) -> ("new picture"=→"new picture":picture)  [unwired: 3 in, 1 out]
